vi "dev_create-2d-gauss.vi"() -> (0 "coordinates":dbl[][](array[numeric]), 1 "StdDev":dbl[](array[numeric]), 2 "Intensity Graph":dbl[][](graph), 3 "Mean":dbl[](array[numeric]), 4 "values":dbl[](array[numeric]))   [LabVIEW 2024]
uses:
  <vilib>/Math Plots/3D Math Plots/3D Contour/3D Contour XCtrl/3D Contour.xctl
  <vilib>/Native 3D Graph/xcontrol/3DPC_SurfacePlot.xctl
  <vilib>/numeric/Random Number (Range) DBL.vi
  <vilib>/Math Plots/3D Math Plots/3D Contour/3D Contour Datatype/Public/Plot Helper (Matrix).vi
  <vilib>/Math Plots/3D Math Plots/3D Contour/3D Contour Datatype/3D Contour Datatype.lvclass
panel:
  out "3D Graph":refnum<class "Base Datatype.lvclass">[](xcontrol)
  out "3D Contour":refnum<class "3D Plot Datatype.lvclass">[](xcontrol)
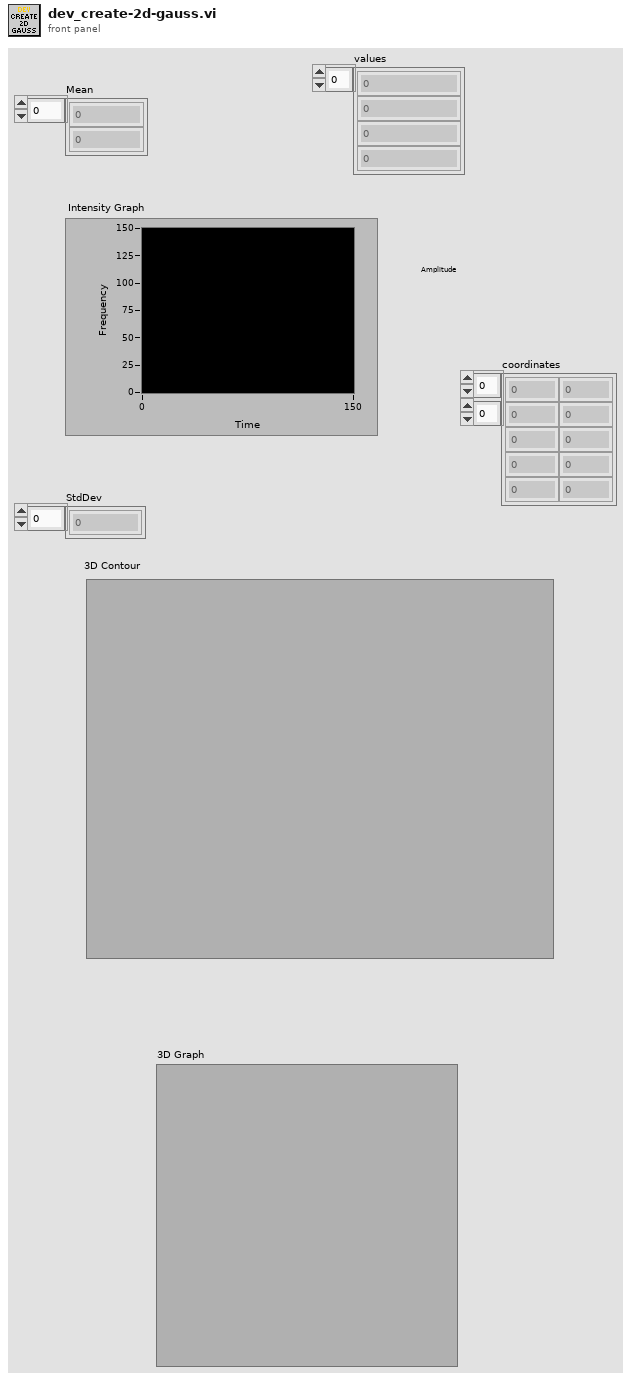
[diagram p1: front panel]
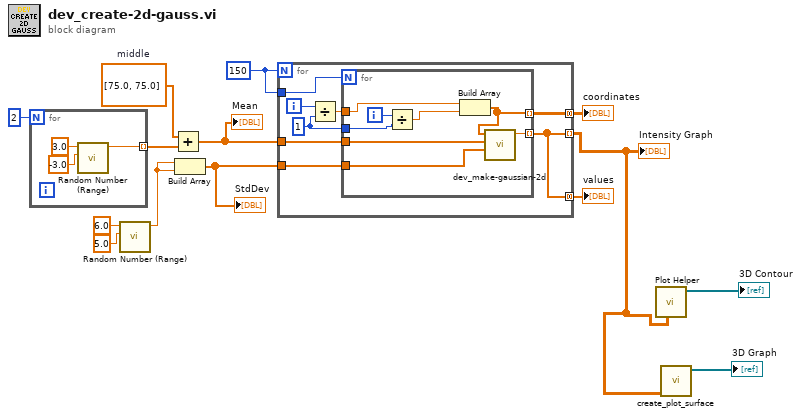
[diagram p0: block diagram]
diagram:
  w14 = dbl[] [75.0, 75.0]  # middle
  w6 = 150
  n1 = for {
    N: 2 -> [_]
    tunnel: [w15] -> w11 mode=indexing
    n2 = call-poly <vilib>:"Random Number (Range).vi"("lower bound (0)"=-3.0, "upper bound (100)"=3.0) -> ("number"=w15:dbl)  [unwired: 9 in]
  }
  n3 = call-poly <vilib>:"Random Number (Range).vi"("lower bound (0)"=5.0, "upper bound (100)"=6.0) -> ("number"=w7:dbl)  [unwired: 9 in]
  n4 = Add(x=w14, y=w11) -> (x+y=w12:dbl[])
  "Mean" <- w12
  n5 = Build Array(w7, w7) -> (w8:dbl[])
  "StdDev" <- w8
  n6 = for {
    N: w6 -> [_]
    tunnel: w8 -> [w25]
    tunnel: [w18] -> w1 mode=indexing
    tunnel: w12 -> [w24]
    tunnel: w6 -> [w23]
    tunnel: [w19] -> w5 mode=concatenating
    tunnel: [w18] -> w4 mode=concatenating
    i -> [w21]
    w20 = 1 ("y")
    n7 = Divide(x=w21, y=w20) -> (x/y=w22:dbl)
    n8 = for {
      N: w23 -> [_]
      tunnel: w25 -> [w33]
      tunnel: [w31] -> w18 mode=indexing
      tunnel: w24 -> [w32]
      tunnel: w22 -> [w30]
      tunnel: w20 -> [w27]
      tunnel: [w26] -> w19 mode=indexing
      i -> [w29]
      n9 = Divide(x=w29, y=w27) -> (x/y=w28:dbl)
      n10 = Build Array(w30, w28) -> (w26:dbl[])
      n11 = call "dev_make-gaussian-2d.vi"("StdDev"=w33, "Mean"=w32, "in"=w26) -> ("out"=w31:dbl)  [unwired: 8 in]
    }
  }
  "Intensity Graph" <- w1
  "coordinates" <- w5
  "values" <- w4
  n12 = call-poly <vilib>:"Plot Helper.vi"("z matrix"=w1) -> ("3D Plot lvclass Array out"=→"3D Contour":refnum<class "3D Plot Datatype.lvclass">[])  [unwired: 5 in, 5 out]
  n13 = call <vilib>:"create_plot_surface.vi"("z matrix"=w1) -> ("plots out"=→"3D Graph":refnum<class "Base Datatype.lvclass">[])  [unwired: 4 in, 6 out]
